vi "Read PID gains.vi"(8 "error in (no error)":errorcluster, 11 "PID in":refnum<class "PID.lvclass">) -> (0 "error out":errorcluster, 2 "PID gains":T1={"proportional gain (Kc)"=1.0, "integral time (Ti, min)"=0.01, "derivative time (Td, min)"=0.0} {"derivative time (Td, min)" format="%.3f"; "integral time (Ti, min)" format="%.3f"; "proportional gain (Kc)" format="%.3f"}, 3 "PID out":refnum<class "PID.lvclass">)   [LabVIEW 2024, in "PID.lvlib" / "PID.lvclass"]
uses:
  PID.lvclass
  PID.lvclass/PID.ctl
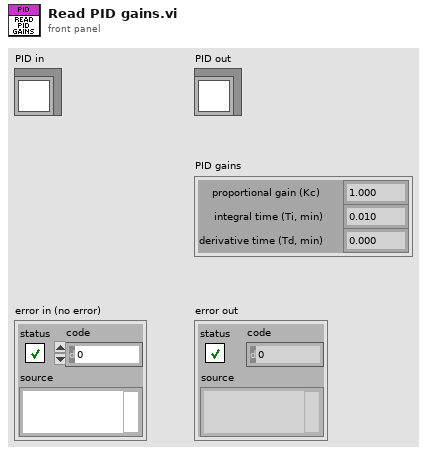
[diagram p1: front panel]
types:
  T1 = cluster{"proportional gain (Kc)":dbl, "integral time (Ti, min)":dbl, "derivative time (Td, min)":dbl}
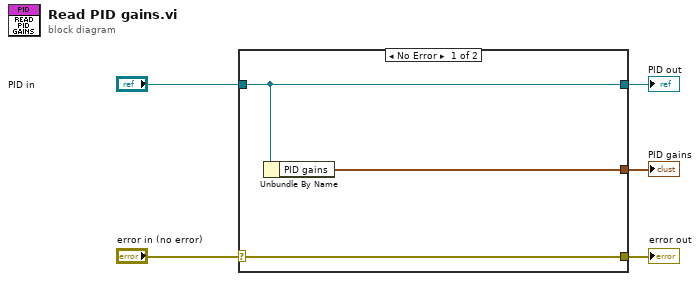
[diagram p0: block diagram]
diagram:
  n1 = case shown="No Error" "error in (no error)" {
    selector: "error in (no error)" -> [w8 w9]
    tunnel: [w8 w9] -> w4
    tunnel: [w7 w10] -> w2
    tunnel: "PID in" -> [w7 w10]
    tunnel: [w6 _] -> w1
    frame No Error {
      n2 = Unbundle By Name(w7) -> ("PID gains"=w6:T1)
    }
    frame Error {
    }
  }
  "error out" <- w4
  "PID out" <- w2
  "PID gains" <- w1
